vi "Banana_Not Equal Value Comparison.vi"(8 "error in (no error)":errorcluster, 9 "Y":variant, 10 "X":variant) -> (0 "error out":errorcluster, 2 "NOT Equal Values?":bool)   [LabVIEW 2021, in "Bananas.lvlib"]
uses:
  <vilib>/Utility/Data Type/Type Definitions/Data Type.ctl
  <vilib>/LabVIEW Open Source Project/Data Manipulation/TypeDescriptor/TypeDescriptor_GetType.vi
  <vilib>/LabVIEW Open Source Project/Data Manipulation/TypeDescriptor/TypeDescriptor_GetName.vi
  <vilib>/LabVIEW Open Source Project/Data Manipulation/TypeDescriptor/TypeDescriptor_GetPString.vi
  <vilib>/LabVIEW Open Source Project/Data Manipulation/Conversions/Flattened nD-Array to Flattened 1D-Array.vi
  Bananas.lvlib
  <vilib>/Utility/Data Type/NI_Data Type.lvlib
  <vilib>/LabVIEW Open Source Project/Data Manipulation/Variant/OpenVariant.lvlib
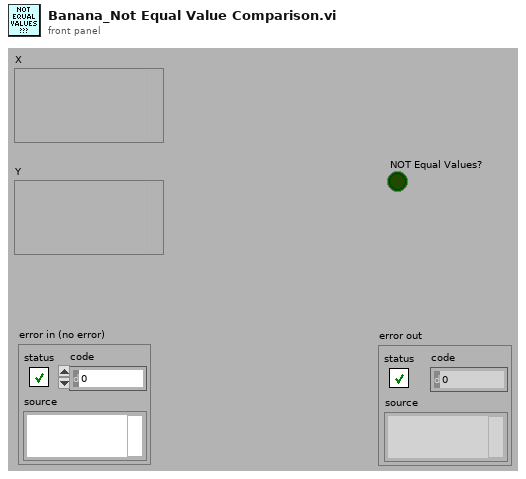
[diagram p1: front panel]
types:
  T1 = typedef "NI_Data Type.lvlib/Data Type.ctl" = enum8{"Invalid Type", "Void", "I8", "I16", "I32", "I64", "U8", "U16", "U32", "U64", "Single Float", "Double Float", "Extended Float", "Single Complex", "Double Complex", "Extended Complex", "Enum U8", "Enum U16", "Enum U32", "Enum U64", "Single Float With Unit", "Double Float With Unit", "Extended Float With Unit", "Single Complex with Unit", "Double Complex with Unit", "Extended Complex with Unit", "Boolean", "String", "Path", "Picture", "Tag", "Array", "Cluster", "Variant", "LV Variant", "Waveform", "Timestamp", "Digital Waveform", "Digital Data", "ExpressData", "Refnum", "External Data", "VI", "Poly VI", "LabVIEW Class Instance", "Fixed Point", "Set Collection", "Map Collection"}
  T2 = typedef "NI_Data Type.lvlib/Unit Info.ctl" = cluster{"Unit Type":T3, "Exponent":i16}
  T3 = typedef "NI_Data Type.lvlib/Unit Type.ctl" = enum16{"Radians", "Steradians", "Seconds", "Meters", "Kilograms", "Amperes", "Kelvins", "Moles", "Candelas", "InvalidUnit"}
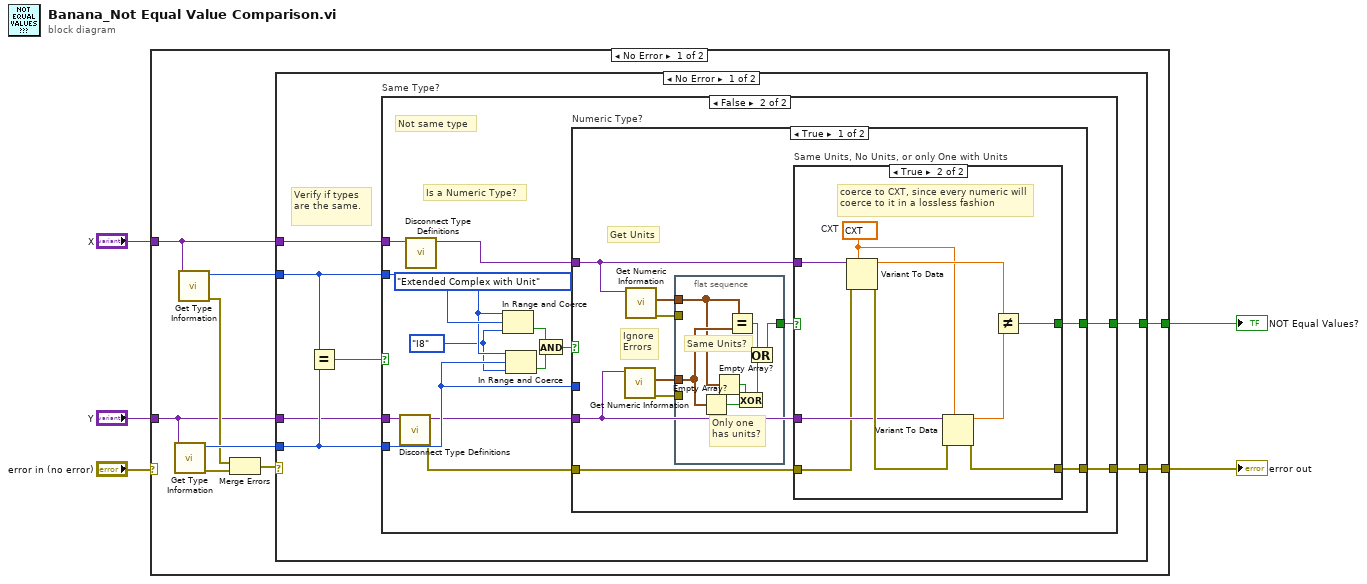
[diagram p0: block diagram]
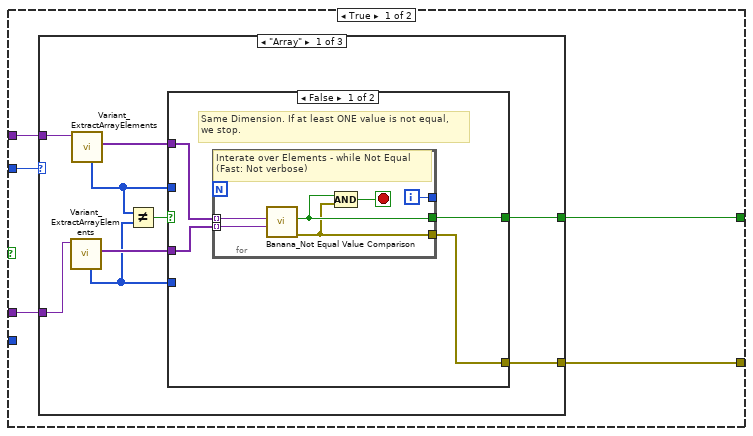
[diagram p2: hidden frame]
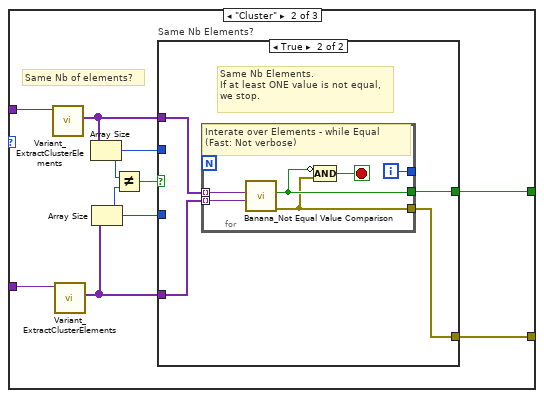
[diagram p4: hidden frame]
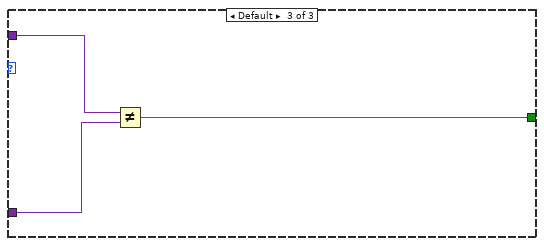
[diagram p6: hidden frame]
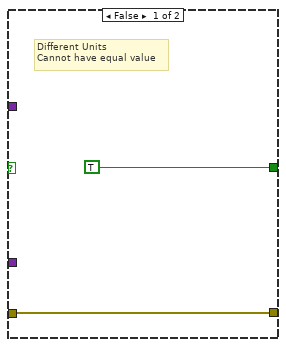
[diagram p7: hidden frame]
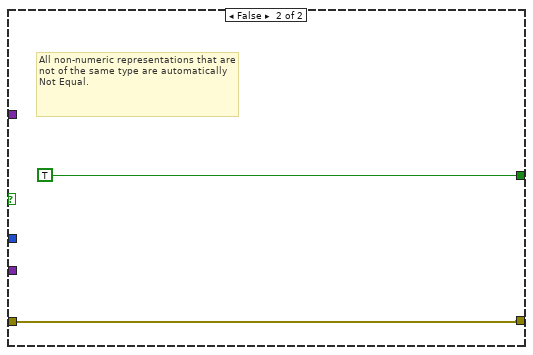
[diagram p8: hidden frame]
diagram:
  n1 = case shown="No Error" "error in (no error)" {
    selector: "error in (no error)" -> [_ w115]
    tunnel: [w14 _] -> w5
    tunnel: [w13 w115] -> w4
    tunnel: "Y" -> [w7 _]
    tunnel: "X" -> [w10 _]
    frame No Error {
      n2 = call <vilib>:"Get Type Information.vi"("variant"=w7) -> ("error out"=w8:errorcluster, "type"=w12:T1)  [unwired: 6 in, 3 out]
      n3 = call <vilib>:"Get Type Information.vi"("variant"=w10) -> ("error out"=w9:errorcluster, "type"=w11:T1)  [unwired: 6 in, 3 out]
      n4 = Merge Errors(w9, w8) -> (w6:errorcluster)
      n5 = case shown="No Error" w6 {
        selector: w6 -> [_ w114]
        tunnel: [w21 _] -> w14
        tunnel: [w20 w114] -> w13
        tunnel: w12 -> [w19 _]
        tunnel: w11 -> [w18 _]
        tunnel: w10 -> [w17 _]
        tunnel: w7 -> [w15 _]
        frame No Error {
          # "Verify if types are the same."
          n6 = Equal?(x=w18, y=w19) -> (x = y?=w16:bool)
          n7 = case "Same Type?" shown="False" w16 {
            tunnel: w17 -> [w24 w76]
            tunnel: w15 -> [w23 w74]
            tunnel: [w26 w77] -> w21
            tunnel: w18 -> [w25 w79]
            tunnel: w19 -> [_ w82]
            tunnel: [w22 w83] -> w20
            frame True {
              n8 = case shown="\"Array\"" w25 {
                tunnel: [w34 w55 w69] -> w26
                tunnel: w24 -> [w30 w50 w68]
                tunnel: w23 -> [w29 w49 w67]
                tunnel: [w35 w54 _] -> w22
                frame "Array" {
                  n9 = call <vilib>:"Variant_ExtractArrayElements.vi"("Array"=w29) -> ("Elements"=w28:variant[], "Dimensions"=w27:u32[])  [unwired: 7 in, 2 out]
                  n10 = call <vilib>:"Variant_ExtractArrayElements.vi"("Array"=w30) -> ("Elements"=w33:variant[], "Dimensions"=w32:u32[])  [unwired: 7 in, 2 out]
                  n11 = Not Equal?(x=w32, y=w27) -> (x != y?=w31:bool)
                  n12 = case shown="False" w31 {
                    selector: w31 -> [_ w46]
                    tunnel: [w36 w46] -> w34
                    tunnel: [w37 _] -> w35
                    tunnel: w32 -> [_ _]
                    tunnel: w27 -> [_ _]
                    tunnel: w33 -> [w39 _]
                    tunnel: w28 -> [w38 _]
                    frame False {
                      # "Same Dimension. If at least ONE value is not equal,\nwe stop."
                      n13 = for {
                        tunnel: w39 -> [w45] mode=indexing
                        tunnel: w38 -> [w44] mode=indexing
                        tunnel: [w43] -> w36
                        tunnel: [w41] -> w37
                        tunnel: [w40] -> _
                        i -> [w40]
                        stop <- w42 stop-if-true
                        # "Interate over Elements - while Not Equal\n(Fast: Not verbose)"
                        n14 = call "Banana_Not Equal Value Comparison.vi"("Y"=w44, "X"=w45) -> ("error out"=w41:errorcluster, "NOT Equal Values?"=w43:bool)  [unwired: 8 in]
                        n15 = Compound Arithmetic op=AND(w43, w41) -> (w42:bool)
                      }
                    }
                    frame True {
                      # "Cannot be equal if dimensions differ"
                    }
                  }
                }
                frame "Cluster" {
                  # "Same Nb of elements?"
                  n16 = call <vilib>:"Variant_ExtractClusterElements.vi"("Cluster"=w50) -> ("Elements"=w48:variant[])  [unwired: 8 in, 2 out]
                  n17 = call <vilib>:"Variant_ExtractClusterElements.vi"("Cluster"=w49) -> ("Elements"=w47:variant[])  [unwired: 8 in, 2 out]
                  n18 = Array Size(array=w48) -> (size(s)=w52:i32)
                  n19 = Array Size(array=w47) -> (size(s)=w51:i32)
                  n20 = Not Equal?(x=w52, y=w51) -> (x != y?=w53:bool)
                  n21 = case "Same Nb Elements?" shown="True" w53 {
                    selector: w53 -> [w56 _]
                    tunnel: [w56 w58] -> w55
                    tunnel: [_ w57] -> w54
                    tunnel: w52 -> [_ _]
                    tunnel: w51 -> [_ _]
                    tunnel: w48 -> [_ w60]
                    tunnel: w47 -> [_ w59]
                    frame False {
                      # "Not Same Nb Elements.\nCannot be equal"
                    }
                    frame True {
                      # "Same Nb Elements. \nIf at least ONE value is not equal,\nwe stop."
                      n22 = for {
                        tunnel: w60 -> [w66] mode=indexing
                        tunnel: w59 -> [w65] mode=indexing
                        tunnel: [w64] -> w58
                        tunnel: [w62] -> w57
                        tunnel: [w61] -> _
                        i -> [w61]
                        stop <- w63 stop-if-true
                        # "Interate over Elements - while Equal\n(Fast: Not verbose)"
                        n23 = call "Banana_Not Equal Value Comparison.vi"("Y"=w65, "X"=w66) -> ("error out"=w62:errorcluster, "NOT Equal Values?"=w64:bool)  [unwired: 8 in]
                        n24 = Compound Arithmetic op=AND(invert w64, w62) -> (w63:bool)
                      }
                    }
                  }
                }
                frame Default {
                  n25 = Not Equal?(x=w68, y=w67) -> (x != y?=w69:bool)
                }
              }
            }
            frame False {
              w71 = Data_Type."I8" ("type")
              w72 = Data_Type."Extended Complex with Unit" ("type")
              # "Not same type"
              # "Is a Numeric Type?"
              n26 = call <vilib>:"Disconnect Type Definitions.vi"("variant in"=w74) -> ("error out"=w70:errorcluster, "variant out"=w73:variant)  [unwired: 9 in]
              n27 = call <vilib>:"Disconnect Type Definitions.vi"("variant in"=w76) -> ("variant out"=w75:variant)  [unwired: 9 in, 1 out]
              n28 = In Range and Coerce(upper limit=w72, x=w79, lower limit=w71) -> (In Range?=w81:bool)  [unwired: 1 out]
              n29 = In Range and Coerce(upper limit=w72, x=w82, lower limit=w71) -> (In Range?=w80:bool)  [unwired: 1 out]
              n30 = And(x=w81, y=w80) -> (x .and. y?=w78:bool)
              n31 = case "Numeric Type?" shown="True" w78 {
                tunnel: w75 -> [w89 _]
                tunnel: w73 -> [w88 _]
                tunnel: w82 -> [_ _]
                tunnel: [w93 TRUE] -> w77
                tunnel: w70 -> [w91 w113]
                tunnel: [w92 w113] -> w83
                frame True {
                  # "Get Units"
                  # "Ignore\nErrors"
                  n32 = call <vilib>:"Get Numeric Information.vi"("variant"=w88) -> ("error out"=w84:errorcluster, "units"=w87:T2[])  [unwired: 7 in, 2 out]
                  n33 = call <vilib>:"Get Numeric Information.vi"("variant"=w89) -> ("error out"=w85:errorcluster, "units"=w86:T2[])  [unwired: 7 in, 2 out]
                  n34 = flat-sequence {
                    tunnel: w86 -> [w110]
                    tunnel: w87 -> [w111]
                    tunnel: [w105] -> w90
                    tunnel: w85 -> [_]
                    tunnel: w84 -> [_]
                    frame #0 {
                      # "Same Units?"
                      # "Only one\nhas units?"
                      n35 = Empty Array?(array=w111) -> (empty?=w109:bool)
                      n36 = Empty Array?(array=w110) -> (empty?=w108:bool)
                      n37 = Equal?(x=w110, y=w111) -> (x = y?=w106:bool)
                      n38 = Exclusive Or(1:w109, 2:w108) -> (0:w107:bool)
                      n39 = Or(x=w106, y=w107) -> (x .or. y?=w105:bool)
                    }
                  }
                  n40 = case "Same Units, No Units, or only One with Units" shown="True" w90 {
                    tunnel: [TRUE w104] -> w93
                    tunnel: [w95 w103] -> w92
                    tunnel: w89 -> [_ w98]
                    tunnel: w88 -> [_ w97]
                    tunnel: w91 -> [w95 w96]
                    frame False {
                      # "Different Units\nCannot have equal value"
                    }
                    frame True {
                      w99 = cxt 0.0+0.0i  # CXT
                      # "coerce to CXT, since every numeric will coerce to it in a lossless fashion"
                      n41 = Variant To Data(error in=w96, type=w99, Variant=w98) -> (data=w102:cxt, error out=w100:errorcluster)
                      n42 = Variant To Data(error in=w100, type=w99, Variant=w97) -> (data=w101:cxt, error out=w103:errorcluster)
                      n43 = Not Equal?(x=w102, y=w101) -> (x != y?=w104:bool)
                    }
                  }
                }
                frame False {
                  # "All non-numeric representations that are not of the same type are automatically Not Equal."
                }
              }
            }
          }
        }
        frame Error {
        }
      }
    }
    frame Error {
    }
  }
  "NOT Equal Values?" <- w5
  "error out" <- w4
